vi "Is Empty Array Variant.vi"(0 "Variant":variant) -> (6 "Variant out":variant, 8 "Empty?":bool)   [LabVIEW 2019, in "HDF5 Tools.lvlib"]
uses:
  HDF5 Tools.lvlib
  <vilib>/Utility/Data Type/NI_Data Type.lvlib
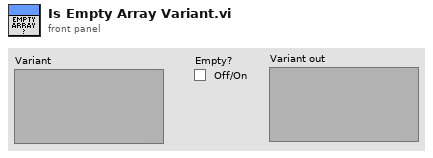
[diagram p1: front panel]
types:
  T1 = typedef "NI_Data Type.lvlib/Data Type.ctl" = enum8{"Invalid Type", "Void", "I8", "I16", "I32", "I64", "U8", "U16", "U32", "U64", "Single Float", "Double Float", "Extended Float", "Single Complex", "Double Complex", "Extended Complex", "Enum U8", "Enum U16", "Enum U32", "Enum U64", "Single Float With Unit", "Double Float With Unit", "Extended Float With Unit", "Single Complex with Unit", "Double Complex with Unit", "Extended Complex with Unit", "Boolean", "String", "Path", "Picture", "Tag", "Array", "Cluster", "Variant", "LV Variant", "Waveform", "Timestamp", "Digital Waveform", "Digital Data", "ExpressData", "Refnum", "External Data", "VI", "Poly VI", "LabVIEW Class Instance", "Fixed Point", "Set Collection", "Map Collection"}
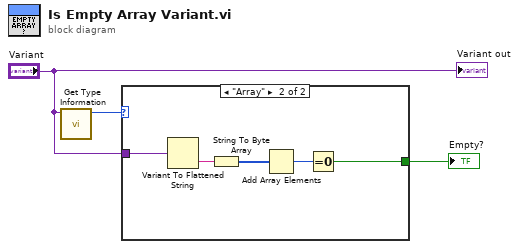
[diagram p0: block diagram]
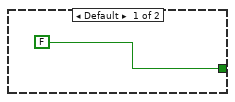
[diagram p2: hidden frame]
diagram:
  n1 = call <vilib>:"Get Type Information.vi"("variant"="Variant") -> ("type"=w3:T1)  [unwired: 6 in, 4 out]
  n2 = case shown="\"Array\"" w3 {
    tunnel: [FALSE w5] -> w2
    tunnel: "Variant" -> [_ w9]
    frame Default {
    }
    frame "Array" {
      n3 = Variant To Flattened String(Variant=w9) -> (data string=w8:string)  [unwired: 1 out]
      n4 = String To Byte Array(string=w8) -> (unsigned byte array=w7:u8[])
      n5 = Add Array Elements(numeric array=w7) -> (sum=w6:u8)
      n6 = Equal To 0?(x=w6) -> (x = 0?=w5:bool)
    }
  }
  "Empty?" <- w2
  "Variant out" <- "Variant"
